vi "SDCP - Serial Port Control.vi"(6 "Command":T1, 7 "VISA resource name":refnum<visa-resource-name>, 8 "error in (no error)":errorcluster, 9 "Transmit bytes":u8[](array[numeric]), 10 "Read byte count":u32, 11 "Baud rate":u32=9600) -> (0 "error out":errorcluster, 1 "Received bytes":u8[](array[numeric]), 2 "Baud rate OUT":u32, 3 "VISA out":refnum<visa-resource-name>)   [LabVIEW 2020]
uses:
  Typedefs/SDCP - Serial Port Control - Commands.ctl
  <vilib>/Instr/_visa.llb/VISA Flush IO Buffer Mask.ctl
  <vilib>/Instr/_visa.llb/VISA Configure Serial Port (Instr).vi
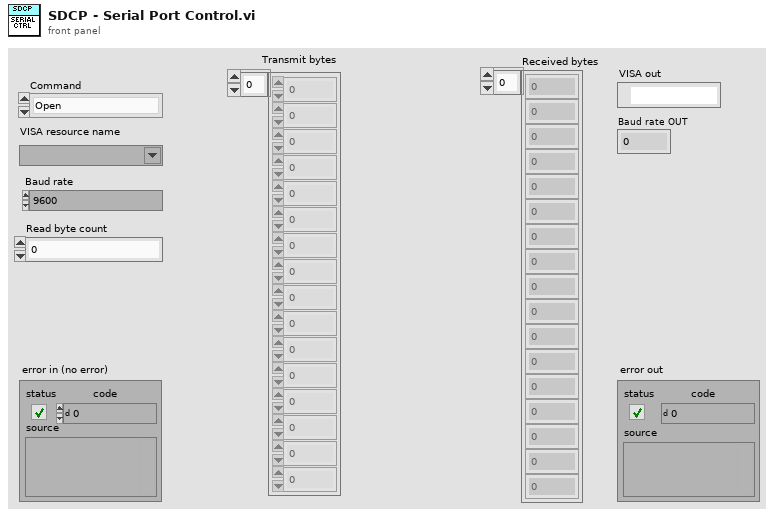
[diagram p1: front panel]
types:
  T1 = typedef "SDCP - Serial Port Control - Commands.ctl" = enum16{"Open", "Read", "Write", "Get instance", "Close"}
  T2 = typedef "VISA Flush IO Buffer Mask.ctl" = u16
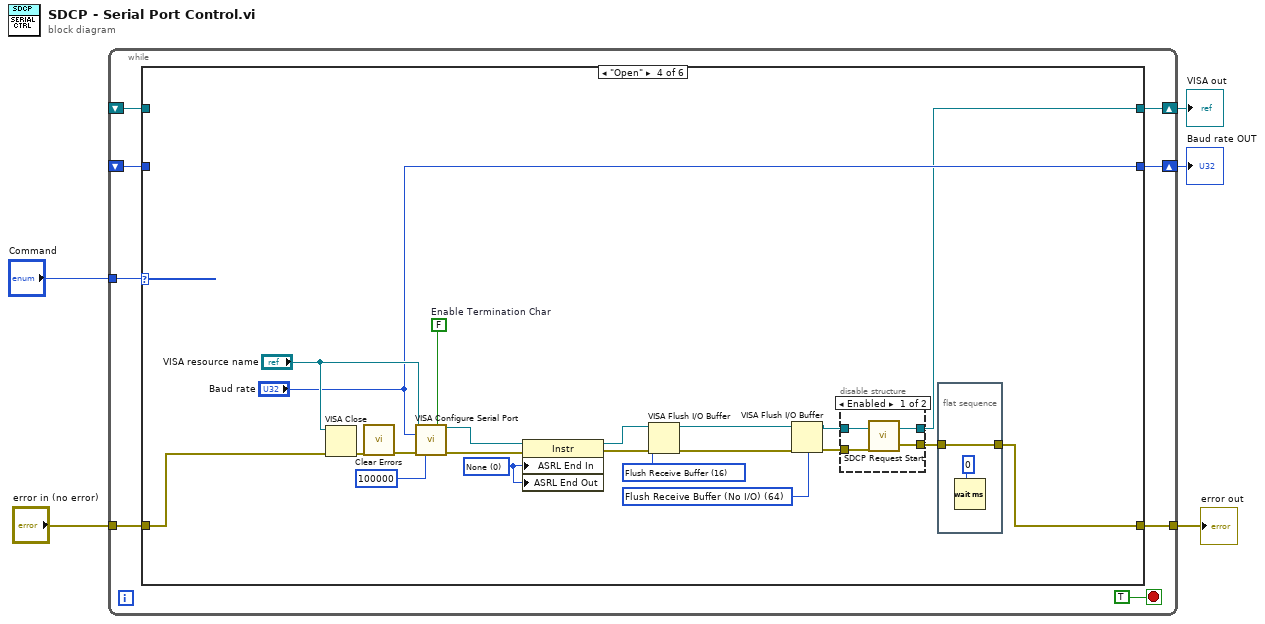
[diagram p0: block diagram]
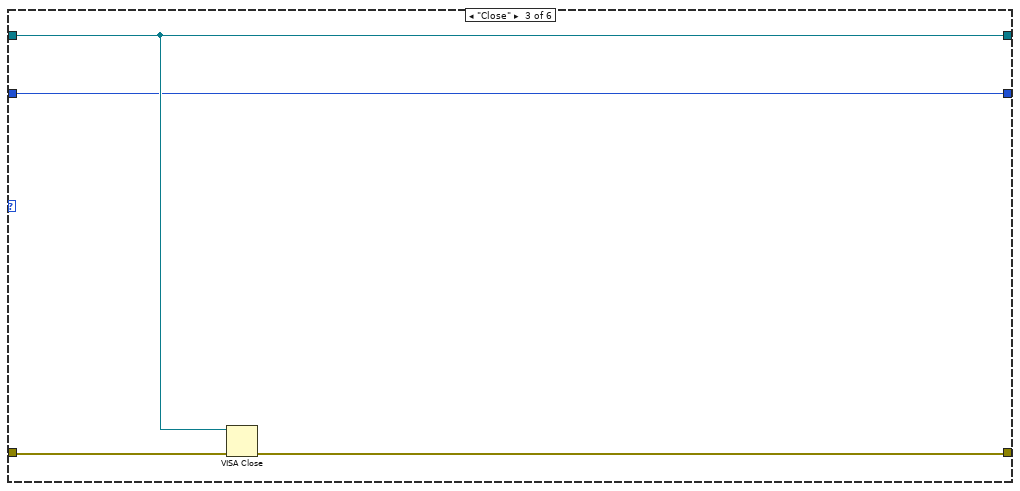
[diagram p4: hidden frame]
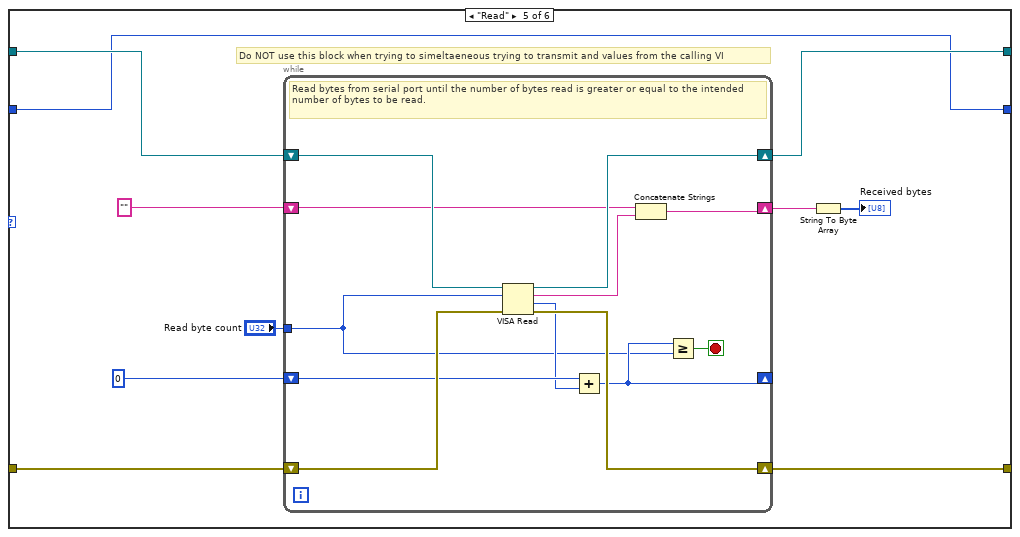
[diagram p6: hidden frame]
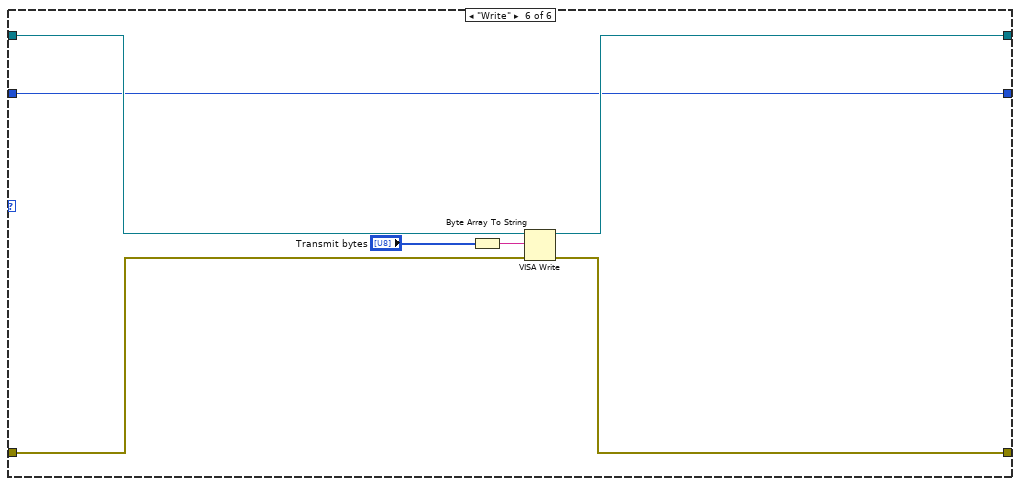
[diagram p7: hidden frame]
diagram:
  n1 = while {
    tunnel: "Command" -> [w11]
    tunnel: "error in (no error)" -> [w12]
    tunnel: [w10] -> w3
    shift-right: [w9] -> w2
    shift-left: _ -> [w8]
    shift-right: [w7] -> w1
    shift-left: _ -> [w6]
    stop <- TRUE stop-if-true
    n2 = case shown="\"Open\"" w11 {
      tunnel: w12 -> [w16 w18 w23 w33 w62 w81]
      tunnel: [w16 w18 w22 w24 w55 w76] -> w10
      tunnel: [w15 w19 w21 w26 w54 w77] -> w9
      tunnel: w8 -> [w15 w19 w21 _ w59 w80]
      tunnel: [w14 w17 w20 "Baud rate" w53 w75] -> w7
      tunnel: w6 -> [w14 w17 w20 _ w53 w75]
      frame Default {
      }
      frame "Get instance" {
      }
      frame "Close" {
        n3 = VISA Close(VISA resource name=w21, error in (no error)=w23) -> (error out=w22:errorcluster)
      }
      frame "Open" {
        w35 = T2 64 items=["Flush Receive Buffer"=16, "Write Transmit Buffer to Device"=32, "Flush Receive Buffer (No I/O)"=64, "Flush Transmit Buffer"=128] ("Mask")
        w38 = T2 16 items=["Flush Receive Buffer"=16, "Write Transmit Buffer to Device"=32, "Flush Receive Buffer (No I/O)"=64, "Flush Transmit Buffer"=128] ("Mask")
        w41 = u16 0 items=["None", "Last Bit", "TermChar"] ("Serial Settings:End Mode for Reads")
        w44 = FALSE  # Enable Termination Char
        n4 = VISA Close(VISA resource name="VISA resource name", error in (no error)=w33) -> (error out=w31:errorcluster)
        n5 = call <vilib>:"Clear Errors.vi"("error in (no error)"=w31) -> ("error out"=w30:errorcluster)  [unwired: 5 in, 1 out]
        n6 = call-poly "VISA Configure Serial Port"("VISA resource name"="VISA resource name", "timeout (10sec)"=u32 100000, "Enable Termination\nChar (T)"=w44, "baud rate (9600)"="Baud rate", "error in (no error)"=w30) -> ("VISA resource name out"=w42:refnum<visa-resource-name>, "error out"=w43:errorcluster)  [unwired: 9 in]
        n7 = property class="Instr"(reference=w42, error in=w43, "ASRL End In"=w41, "ASRL End Out"=w41) -> (reference out=w39:refnum<visa-resource-name>, error out=w40:errorcluster)
        n8 = VISA Flush I/O Buffer(VISA resource name=w39, mask (16)=w38, error in (no error)=w40) -> (VISA resource name out=w36:refnum<visa-resource-name>, error out=w37:errorcluster)
        n9 = VISA Flush I/O Buffer(VISA resource name=w36, mask (16)=w35, error in (no error)=w37) -> (VISA resource name out=w28:refnum<visa-resource-name>, error out=w27:errorcluster)
        n10 = disable-structure shown="Enabled" {
          disable-tunnel: w28 -> [w50 w52]
          disable-tunnel: w27 -> [w49 w51]
          disable-tunnel: [w48 w52] -> w26
          disable-tunnel: [w47 w51] -> w25
          frame Enabled {
            n11 = call "SDCP Request Start.vi"("error in (no error)"=w49, "COM Port"=w50) -> ("error out"=w47:errorcluster, "COM Port Out"=w48:refnum<visa-resource-name>)
          }
          frame Disabled {
          }
        }
        n12 = flat-sequence {
          tunnel: w25 -> [w46]
          tunnel: [w46] -> w24
          frame #0 {
            n13 = Wait (ms)(milliseconds to wait=u32 0) -> ()  [unwired: 1 out]
          }
        }
      }
      frame "Read" {
        # "Do NOT use this block when trying to simeltaeneous trying to transmit and values from the calling VI"
        n14 = while {
          shift-right: [w73] -> w55
          shift-left: w62 -> [w74]
          tunnel: "Read byte count" -> [w64]
          shift-right: [w65] -> _
          shift-left: u32 0 -> [w70]
          shift-right: [w71] -> w54
          shift-left: w59 -> [w72]
          shift-right: [w66] -> w57
          shift-left: "" -> [w68]
          stop <- w63 stop-if-true
          # "Read bytes from serial port until the number of bytes read is greater or equal to the intended number of bytes to be read."
          n15 = VISA Read(VISA resource name=w72, byte count=w64, error in (no error)=w74) -> (VISA resource name out=w71:refnum<visa-resource-name>, read buffer=w67:string, return count=w69:u32, error out=w73:errorcluster)
          n16 = Add(x=w70, y=w69) -> (x+y=w65:u32)
          n17 = Concatenate Strings(w68, w67) -> (w66:string)
          n18 = Greater Or Equal?(x=w65, y=w64) -> (x >= y?=w63:bool)
        }
        n19 = String To Byte Array(string=w57) -> (unsigned byte array=→"Received bytes":u8[])
      }
      frame "Write" {
        n20 = Byte Array To String(unsigned byte array="Transmit bytes") -> (string=w79:string)
        n21 = VISA Write(VISA resource name=w80, write buffer=w79, error in (no error)=w81) -> (VISA resource name out=w77:refnum<visa-resource-name>, error out=w76:errorcluster)  [unwired: 1 out]
      }
    }
  }
  "error out" <- w3
  "VISA out" <- w2
  "Baud rate OUT" <- w1
